vi "SendToGserver.vi"(7 "Query_type":T1, 8 "error in (no error)":errorcluster, 9 "data":variant, 10 "Address":string, 11 "FAMM in":refnum<class "FAMM.lvclass">) -> (0 "error out":errorcluster, 3 "FAMM out":refnum<class "FAMM.lvclass">)   [LabVIEW 2020, in "Sgraph_lib_V1.lvlib" / "FAMM.lvclass"]
doc: "Andre Koelewijn, 17 jan 2021\n\nReturn data to Gserver.\nThe address is meant to indicatie for which Gviewer instance this data should be parsed."
uses:
  FAMM.lvclass
  Gserver/controls/Typedef_QueryType.ctl
  Gserver/controls/Typedef_Gviewer-Query.ctl
  FAMM.lvclass/FAMM.ctl
  Gserver/Gserver.lvclass
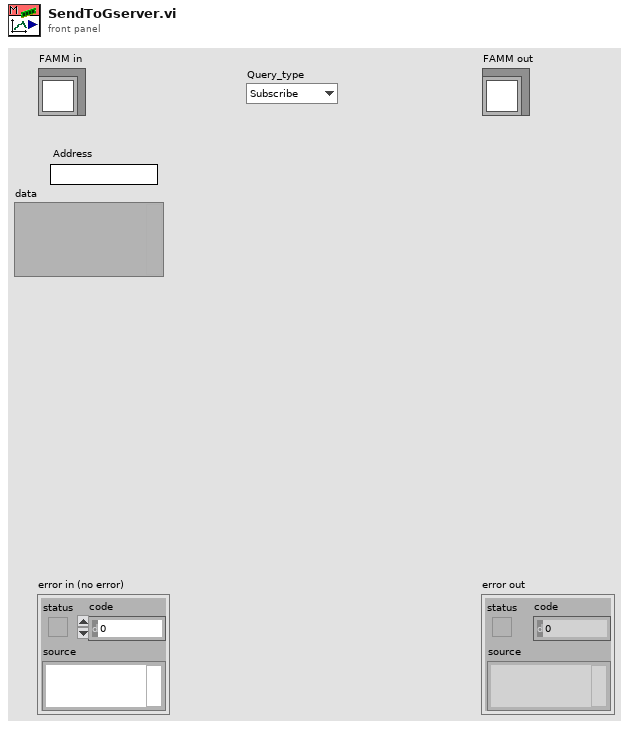
[diagram p1: front panel]
types:
  T1 = typedef "Sgraph_lib_V1.lvlib/Gserver.lvclass/Typedef_QueryType.ctl" = enum16{"Subscribe", "DataRequest", "RequestAllTags", "RequestIniPath", "FAMMstarted", "SetClientOptions", "GviewerUpdate", "OpenNewGraph", "CloseClient", "CloseAllClients", "Close Gserver", "OpenMemoryMap", "MeMapDataRequest", "MeMapDataResponse", "OpenDBeditor", "CheckDBeditorRunning", "StoppedDBeditor", "SaveDB_TAGpropRecord", "ConfirmDB_TAGpropSave"}
  T2 = typedef "Sgraph_lib_V1.lvlib/Gserver.lvclass/Typedef_Gviewer-Query.ctl" = cluster{"Query_type":T1, "data":variant, "Source":string, "Time Stamp":timestamp}
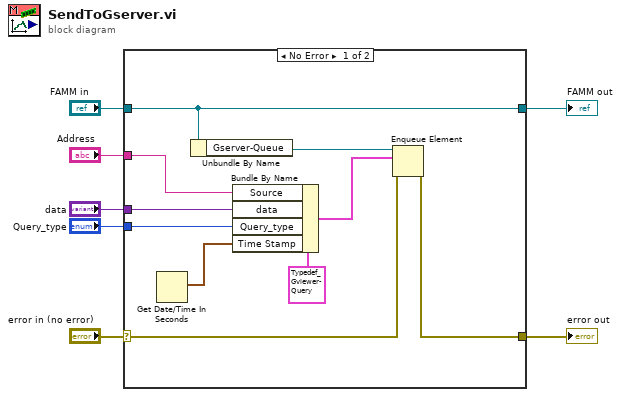
[diagram p0: block diagram]
diagram:
  n1 = case shown="No Error" "error in (no error)" {
    selector: "error in (no error)" -> [w15 w19]
    tunnel: [w14 w19] -> w6
    tunnel: [w17 w18] -> w4
    tunnel: "FAMM in" -> [w17 w18]
    tunnel: "Address" -> [w12 _]
    tunnel: "data" -> [w10 _]
    tunnel: "Query_type" -> [w9 _]
    frame No Error {
      n2 = Get Date/Time In Seconds() -> (seconds since 1Jan1904=w8:timestamp)
      n3 = Unbundle By Name(w17) -> ("Gserver-Queue"=w16:refnum<queue>)
      n4 = Bundle By Name(cluster=T2 {"Query_type"=enum."Subscribe", "data"=variant, "Source"="", "Time Stamp"=timestamp(0 s since 1904-01-01)} ("element"), "Source"=w12, "data"=w10, "Query_type"=w9, "Time Stamp"=w8) -> (w11:T2)
      n5 = Enqueue Element(queue=w16, element=w11, error in (no error)=w15) -> (error out=w14:errorcluster)  [unwired: 1 in, 2 out]
    }
    frame Error {
    }
  }
  "error out" <- w6
  "FAMM out" <- w4
